vi "TDMSFileGen.vi"(8 "error in (no error)":errorcluster, 11 "Who is doing the test?":string) -> (0 "error out":errorcluster, 3 "appended path":path)   [LabVIEW 2019]
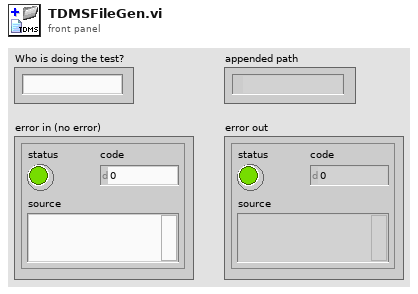
[diagram p1: front panel]
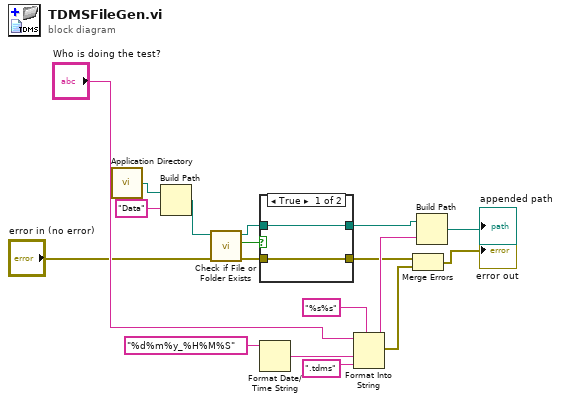
[diagram p0: block diagram]
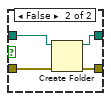
[diagram p2: hidden frame]
diagram:
  n1 = call <vilib>:"Application Directory.vi"() -> ("Application Directory"=w1:path)
  n2 = Build Path(base path=w1, name or relative path="Data") -> (appended path=w7:path)
  n3 = call <vilib>:"Check if File or Folder Exists.vi"("error in (no error)"="error in (no error)", "path"=w7) -> ("error out"=w11:errorcluster, "file or folder exists?"=w9:bool, "dup path"=w10:path)  [unwired: 7 in]
  n4 = case shown="True" w9 {
    tunnel: [w20 w24] -> w16
    tunnel: w10 -> [w20 w23]
    tunnel: w11 -> [w19 w22]
    tunnel: [w19 w21] -> w13
    frame True {
    }
    frame False {
      n5 = Create Folder(path (use dialog)=w23, error in=w22) -> (created path=w24:path, error out=w21:errorcluster)  [unwired: 1 in, 1 out]
    }
  }
  n6 = Format Date/Time String(time format string (%c)="%d%m%y_%H%M%S") -> (date/time string=w3:string)  [unwired: 2 in]
  n7 = Format Into String(format string="%s%s", initial string="Who is doing the test?", w3, ".tdms" ("input 2")) -> (resulting string=w15:string, error out=w12:errorcluster)  [unwired: 1 in]
  n8 = Merge Errors(w13, w12) -> (→"error out":errorcluster)
  n9 = Build Path(base path=w16, name or relative path=w15) -> (appended path=→"appended path":path)
